vi "VI Tree.vi"   [LabVIEW 2018, in "Queue.lvlib"]
uses:
  Queue.lvlib
  16166754-5e17-4172-8fef-04d17df9ff6d.vi
  419261d6-cfd9-4367-a5e7-292623275988.vi
  47078371-e51e-4a35-a069-06550877b838.vi
  b288d960-20d2-4226-b72b-ebf4ce870cf4.vi
  d27c39a2-1da4-4b9d-956b-67a2f9c394d0.vi
  d46e186b-37ef-4304-986d-5c6bda912150.vi
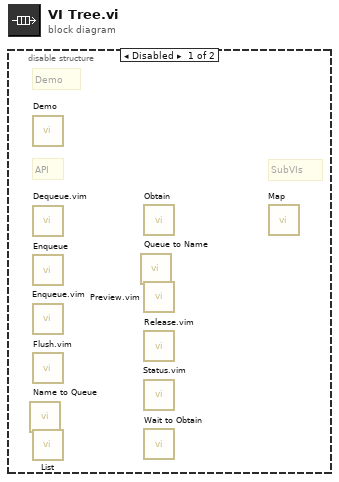
[diagram p0: block diagram]
diagram:
  n1 = disable-structure shown="Disabled" {
    frame Disabled {
      # "SubVIs"
      # "API"
      # "Demo"
      n2 = call "Name to Queue.vi"() -> ()  [unwired: 8 in, 2 out]
      n3 = call "Demo.vi"() -> ()  [unwired: 12 in]
      n4 = call "Dequeue.vim"() -> ()  [unwired: 6 in, 6 out]
      n5 = call "Enqueue.vi"() -> ()  [unwired: 10 in, 2 out]
      n6 = call "Enqueue.vim"() -> ()  [unwired: 10 in, 2 out]
      n7 = call "Flush.vim"() -> ()  [unwired: 7 in, 5 out]
      n8 = call "List.vi"() -> ()  [unwired: 9 in, 3 out]
      n9 = call "Queue to Name.vi"() -> ()  [unwired: 8 in, 2 out]
      n10 = call "Obtain.vi"() -> ()  [unwired: 9 in, 3 out]
      n11 = call "Preview.vim"() -> ()  [unwired: 6 in, 6 out]
      n12 = call "Release.vim"() -> ()  [unwired: 9 in, 3 out]
      n13 = call "Status.vim"() -> ()  [unwired: 4 in, 8 out]
      n14 = call "Wait to Obtain.vi"() -> ()  [unwired: 9 in, 3 out]
      n15 = call "Map.vi"() -> ()  [unwired: 10 in, 2 out]
    }
    frame Enabled {
    }
  }
